vi "switch_counter.vi"() -> ()   [LabVIEW 2014]
panel:
  in  "Step Name":u16(ring) items=["Step 0", "Step 1", "Step 2", "Step 3"]
  in  "stop":bool
  out "Numeric":dbl
  in  "Boolean 4":bool
  in  "Boolean 3":bool
  in  "Boolean 2":bool
  in  "Boolean":bool
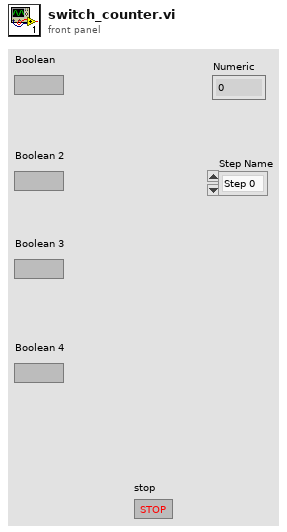
[diagram p1: front panel]
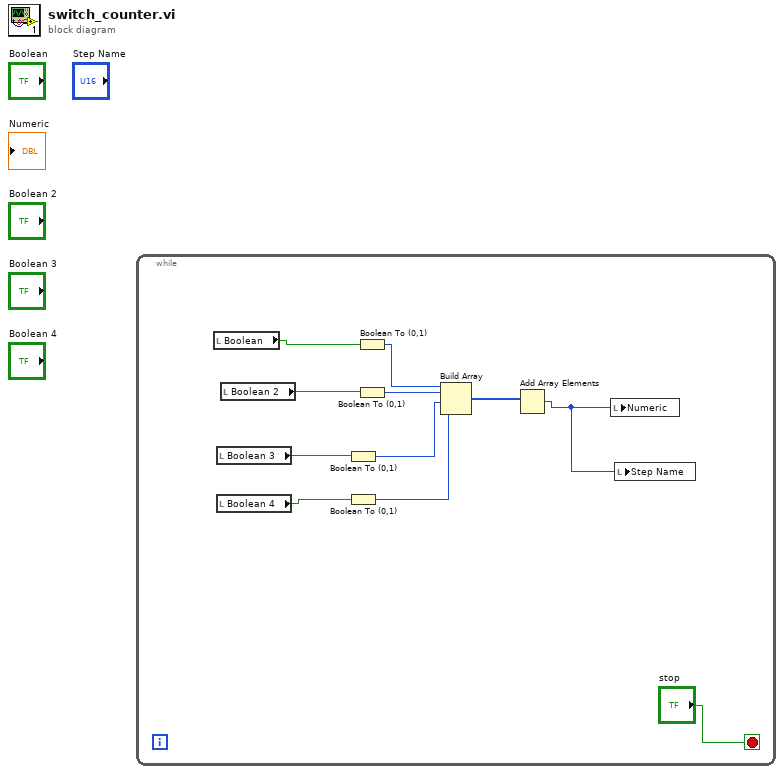
[diagram p0: block diagram]
diagram:
  n1 = while {
    stop <- "stop" stop-if-true
    n2 = local read "Boolean"() -> (w10:bool)
    n3 = local read "Boolean 3"() -> (w8:bool)
    n4 = local read "Boolean 4"() -> (w7:bool)
    n5 = local read "Boolean 2"() -> (w9:bool)
    n6 = Boolean To (0,1)(Boolean=w8) -> (0, 1=w4:i16)
    n7 = Boolean To (0,1)(Boolean=w7) -> (0, 1=w3:i16)
    n8 = Boolean To (0,1)(Boolean=w10) -> (0, 1=w6:i16)
    n9 = Boolean To (0,1)(Boolean=w9) -> (0, 1=w5:i16)
    n10 = Build Array(w6, w5, w4, w3) -> (w2:i16[])
    n11 = Add Array Elements(numeric array=w2) -> (sum=w1:i16)
    n12 = local write "Numeric"(w1) -> ()
    n13 = local write "Step Name"(w1) -> ()
  }
